vi "Add Log Entry.vi"(8 "error in (no error)":errorcluster, 9 "Message":string, 10 "From (SERVER)":string="SERVER", 11 "LV Chat Server in":refnum<class "LV Chat Server.lvclass">) -> (0 "error out":errorcluster, 3 "LV Chat Server out":refnum<class "LV Chat Server.lvclass">)   [LabVIEW 2020, in "LV Chat Server.lvclass"]
uses:
  LV Chat Server.lvclass
  Log Event Data.ctl
  Data Types/Message.ctl
  LV Chat Server.lvclass/LV Chat Server.ctl
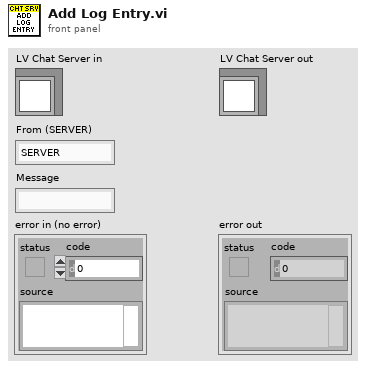
[diagram p1: front panel]
types:
  T1 = typedef "LV Chat Server.lvclass/Log Event Data.ctl" = cluster{"Item":T2}
  T2 = typedef "Message.ctl" = cluster{"From":string, "Time":dbl, "Message":string}
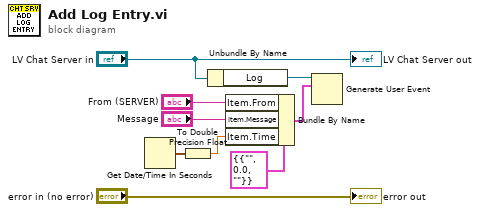
[diagram p0: block diagram]
diagram:
  n1 = Get Date/Time In Seconds() -> (seconds since 1Jan1904=w5:timestamp)
  n2 = To Double Precision Float(number=w5) -> (double precision float=w4:dbl)
  n3 = Unbundle By Name("LV Chat Server in") -> ("Log"=w2:refnum<user-event>)
  n4 = Bundle By Name(cluster=T1 {"Item"={"From"="", "Time"=0.0, "Message"=""}} ("Log Event Data"), "Item.From"="From (SERVER)", "Item.Message"="Message", "Item.Time"=w4) -> (w1:T1)
  n5 = Generate User Event(user event=w2, event data cluster=w1) -> ()  [unwired: 2 in, 2 out]
  "error out" <- "error in (no error)"
  "LV Chat Server out" <- "LV Chat Server in"
